vi "Countdown.vi"(1 "Autosequence Start":bool, 2 "Time Until Hotfire":dbl, 3 "Shift Register In":dbl, 4 "Iteration Time":u32) -> (5 "T Minus":dbl, 6 "Shift Register Out":dbl)   [LabVIEW 2024]
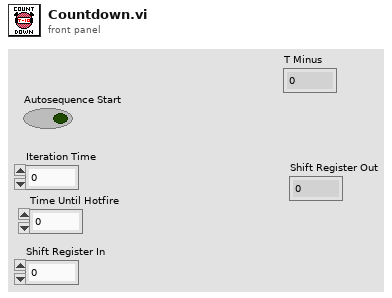
[diagram p1: front panel]
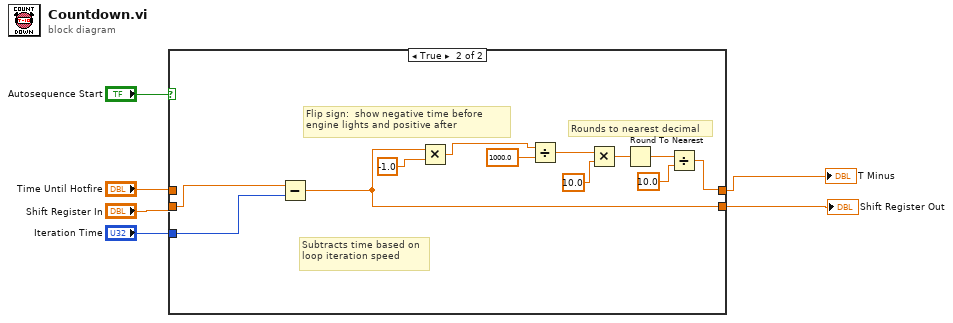
[diagram p0: block diagram]
diagram:
  n1 = case shown="True" "Autosequence Start" {
    tunnel: "Iteration Time" -> [_ w12]
    tunnel: "Time Until Hotfire" -> [w7 _]
    tunnel: [w7 w16] -> w1
    tunnel: "Shift Register In" -> [w8 w15]
    tunnel: [w8 w14] -> w2
    frame False {
    }
    frame True {
      # "Flip sign:  show negative time before engine lights and positive after"
      # "Rounds to nearest decimal"
      # "Subtracts time based on loop iteration speed"
      n2 = Subtract(x=w15, y=w12) -> (x-y=w14:dbl)
      n3 = Multiply(x=w14, y=-1.0) -> (x*y=w10:dbl)
      n4 = Divide(x=w10, y=1000.0) -> (x/y=w9:dbl)
      n5 = Multiply(x=w9, y=10.0) -> (x*y=w20:dbl)
      n6 = Round To Nearest(number=w20) -> (nearest integer value=w18:dbl)
      n7 = Divide(x=w18, y=10.0) -> (x/y=w16:dbl)
    }
  }
  "Shift Register Out" <- w2
  "T Minus" <- w1
